vi "VciEnumDeviceReset.vi"(3 "error in":errorcluster {"code" format="%.0x"}, 5 "Enum Handle in":u32 format="%x") -> (0 "error out":errorcluster {"code" format="%.0x"}, 2 "Enum Handle out":u32)   [LabVIEW 2011]
doc: "Resets the VCI device enumerator."
uses:
  vcilva.dll
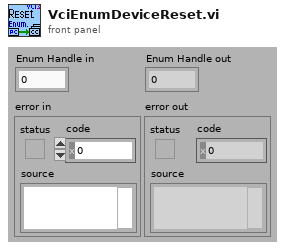
[diagram p1: front panel]
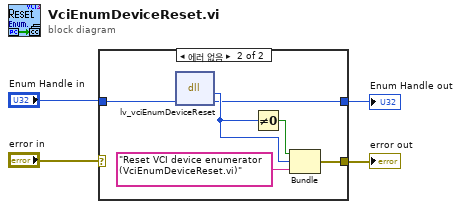
[diagram p0: block diagram]
diagram:
  n1 = case shown="에러 없음" "error in" {
    selector: "error in" -> [w6 _]
    tunnel: [w6 w12] -> w3
    tunnel: "Enum Handle in" -> [w5 w8]
    tunnel: [w5 w7] -> w1
    frame Error {
    }
    frame No Error {
      n2 = dll-call lib="vcilva.dll" fn="lv_vciEnumDeviceReset"("hEnum"=w8) -> (w9:i32, "hEnum"=w7:u32)  [unwired: 3 in, 2 out]
      n3 = Not Equal To 0?(x=w9) -> (x != 0?=w11:bool)
      n4 = Bundle(w11, w9, "Reset VCI device enumerator (VciEnumDeviceReset.vi)") -> (w12:errorcluster)  [unwired: 1 in]
    }
  }
  "error out" <- w3
  "Enum Handle out" <- w1
